vi "H5FileStoreTest.vi"() -> ()   [LabVIEW 2020]
uses:
  <vilib>/UPVI/lvhdf5/file.llb/LVH5F Operation.ctl
  <vilib>/UPVI/lvhdf5/dataset.llb/LVH5D Operation.ctl
  <vilib>/Utility/miscctls.llb/LVRectTypeDef.ctl
  <vilib>/UPVI/lvhdf5/attribute.llb/LVH5A Operation.ctl
  <vilib>/UPVI/lvhdf5/group.llb/H5G_obj_t.ctl
  <vilib>/UPVI/lvhdf5/identifier.llb/Not an HDF5 Refnum Constant.vi
  <vilib>/UPVI/lvhdf5/common.llb/To HDF5 Ref.vi
  <vilib>/UPVI/lvhdf5/utility.llb/Select HDF5 Dialog.vi
  <vilib>/UPVI/lvhdf5/utility.llb/Select HDF5 Dialog (Object Only).vi
  <vilib>/UPVI/lvhdf5/dataset.llb/Simple H5Dwrite (Variant).vi
  <vilib>/UPVI/lvhdf5/attribute.llb/Write Multiple Attributes.vi
  <vilib>/UPVI/lvhdf5/dataset.llb/H5Dclose.vi
  <vilib>/UPVI/lvhdf5/dataset.llb/Write Dataset with Attributes.xnode
  <vilib>/UPVI/lvhdf5/library.llb/HDF5 Ref.ctl
  <vilib>/Utility/error.llb/Error Cluster From Error Code.vi
  <vilib>/UPVI/lvhdf5/dataset.llb/OpenCreateReplace Dataset by Element Type.vi
  <vilib>/UPVI/lvhdf5/dataspace.llb/H5Sselect_hyperslab.vi
  <vilib>/UPVI/lvhdf5/dataset.llb/H5Dwrite (Variant).vi
  <vilib>/UPVI/lvhdf5/dataset.llb/H5Dget_space.vi
  <vilib>/UPVI/lvhdf5/attribute.llb/private/LVH5AwriteWDTAttrs.vi
  <vilib>/UPVI/lvhdf5/dataspace.llb/H5Sclose.vi
  <vilib>/UPVI/lvhdf5/utility.llb/Select HDF5 Dialog (File and Object).vi
  <vilib>/Utility/VariantDataType/GetClusterInfo.vi
  <vilib>/Utility/VariantDataType/VariantType.lvlib
  <vilib>/Utility/VariantDataType/GetTypeInfo.vi
  <vilib>/UPVI/lvhdf5/attribute.llb/Cluster to Attribute Array.xnode
panel:
  in  "path":path
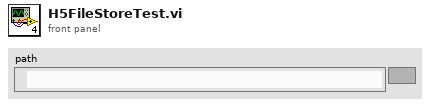
[diagram p1: front panel]
types:
  T1 = typedef "LVH5D Operation.ctl" = enum16{"open", "replace", "create", "open or create", "create or replace", "create or replace with confirmation"}
  T2 = typedef "LVH5F Operation.ctl" = enum16{"open", "open or create", "create or replace", "create or replace (with confirmation)", "create", "open (read only)"}
  T3 = typedef "HDF5 Ref.ctl" = refnum<k1>
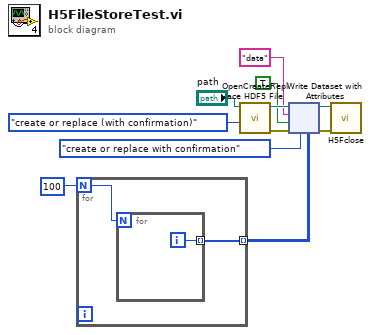
[diagram p0: block diagram]
diagram:
  n1 = for {
    N: 100 -> [w12]
    tunnel: [w13] -> w4 mode=indexing
    n2 = for {
      N: w12 -> [_]
      tunnel: [w14] -> w13 mode=indexing
      i -> [w14]
    }
  }
  n3 = call <vilib>:"OpenCreateReplace HDF5 File.vi"("function (open or create)"=LVH5F_Operation."create or replace (with confirmation)", "path"="path") -> ("error out"=w6:errorcluster, "HDF5 Ref out"=w9:T3)  [unwired: 6 in]
  n4 = xnode "Write Dataset with Attributes"("Dataset Path"="data", "Unlimited  dataset (F)"=TRUE, "error in (no error)"=w6, "operation (open or create)"=LVH5D_Operation."create or replace with confirmation", "HDF5 Path or Ref"=w9, "Data"=w4) -> ("HDF5 Ref out"=w2:T3, "error out"=w1:errorcluster)  [unwired: 2 in, 1 out]
  n5 = call <vilib>:"H5Fclose.vi"("error in (no error)"=w1, "HDF5 Ref"=w2) -> ()  [unwired: 7 in, 1 out]
